vi "Test_ReadActiveItem_RetrieveItem.vi"(8 "error in (no error)":errorcluster, 11 "TestCase in":refnum<class "TestStringList.lvclass">) -> (0 "error out":errorcluster, 3 "TestCase out":refnum<class "TestStringList.lvclass">)   [LabVIEW 2015, in "StringList.lvlib" / "TestStringList.lvclass"]
uses:
  TestStringList.lvclass
  <vilib>/addons/_JKI Toolkits/VI Tester/TestCase.llb/TestCase.lvclass
  StringList.lvclass
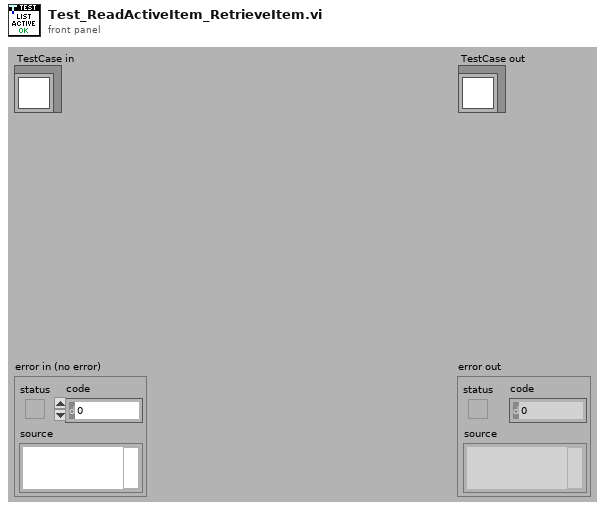
[diagram p1: front panel]
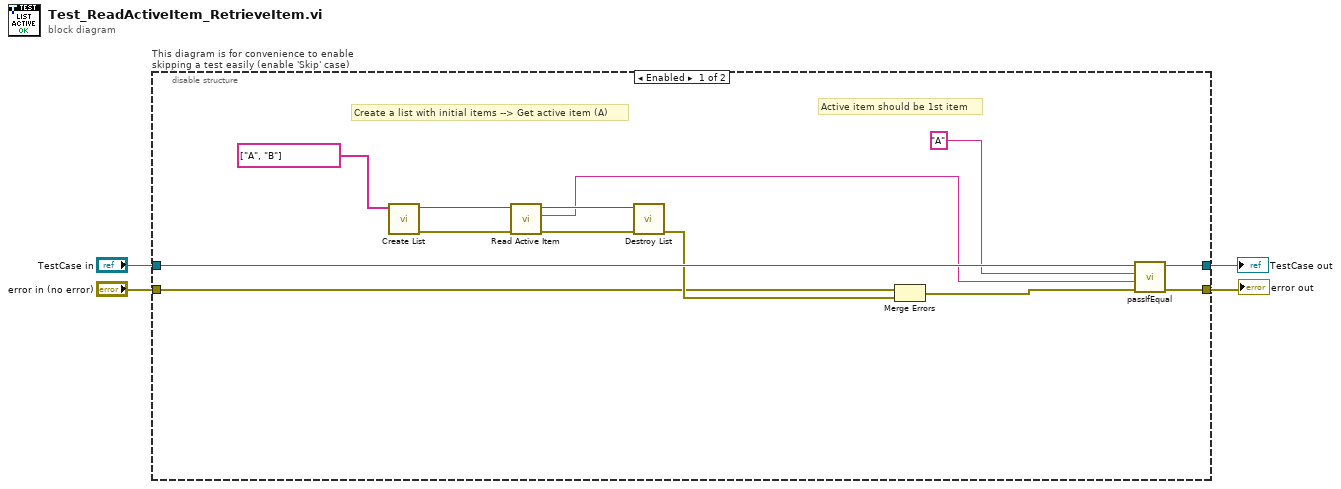
[diagram p0: block diagram]
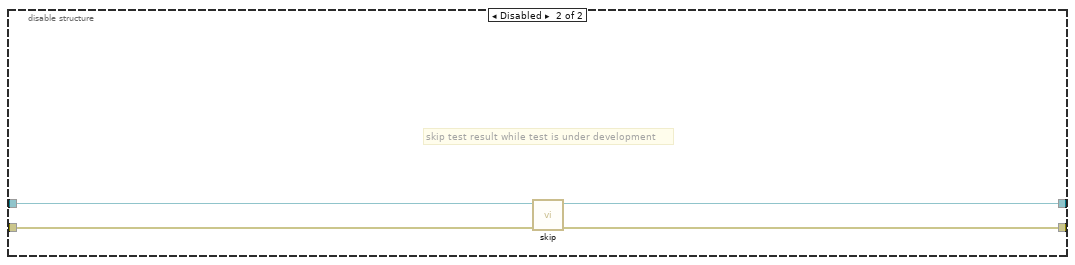
[diagram p2: hidden frame]
diagram:
  n1 = disable-structure "This diagram is for convenience to enable skipping a test easily (enable 'Skip' case)" shown="Enabled" {
    disable-tunnel: "TestCase in" -> [w17 w21]
    disable-tunnel: [w16 w19] -> w1
    disable-tunnel: [w15 w20] -> w3
    disable-tunnel: "error in (no error)" -> [w12 w18]
    frame Enabled {
      # "Active item should be 1st item"
      # "Create a list with initial items --> Get active item (A)"
      n2 = call "Create List.vi"("Initial Strings (empty list)"=string[] ["A", "B"]) -> ("error out"=w8:errorcluster, "StringList Reference"=w11:refnum<data-value>)  [unwired: 9 in]
      n3 = call "Read Active Item.vi"("error in (no error)"=w8, "StringList Reference"=w11) -> ("error out"=w7:errorcluster, "Item"=w6:string, "StringList Reference"=w9:refnum<data-value>)  [unwired: 7 in]
      n4 = call "Destroy List.vi"("error in (no error)"=w7, "StringList Reference"=w9) -> ("error out"=w13:errorcluster)  [unwired: 8 in, 1 out]
      n5 = Merge Errors(w12, w13) -> (w14:errorcluster)
      n6 = call-dynamic "passIfEqual.vi"("error in (no error)"=w14, "y"=w6, "x"="A", "TestCase in"=w17) -> ("error out"=w15:errorcluster, "TestCase out"=w16:refnum<class "TestStringList.lvclass">)  [unwired: 6 in]
    }
    frame Disabled {
      # "skip test result while test is under development"
      n7 = call <vilib>:"skip.vi"("error in (no error)"=w18, "TestCase in"=w21) -> ("error out"=w20:errorcluster, "TestCase out"=w19:refnum<class "TestStringList.lvclass">)  [unwired: 8 in]
    }
  }
  "error out" <- w3
  "TestCase out" <- w1
